vi "Lognormal Moments.vi"(9 "c":dbl=0.6, 10 "b":dbl=1.0) -> (0 "error":i32, 2 "variance":dbl=0.6211037960835473, 3 "mean":dbl=1.1972173631218102)   [LabVIEW 2017, in "NI_Gmath.lvlib"]
doc: "Returns the expected mean and variance of the random variate X, where X describes the selected distribution type. You must manually select the polymorphic instance to use."
uses:
  NI_Gmath.lvlib
  st_error_code.ctl
panel:
  # "Lognormal Moments"
  # "median (scale)"
  # "standard dev (shape)"
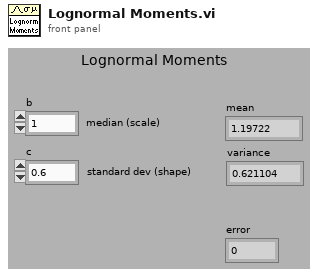
[diagram p1: front panel]
types:
  T1 = typedef "NI_Gmath.lvlib/st_error_code.ctl" = i32
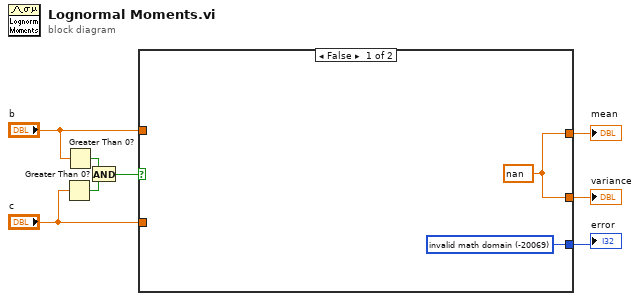
[diagram p0: block diagram]
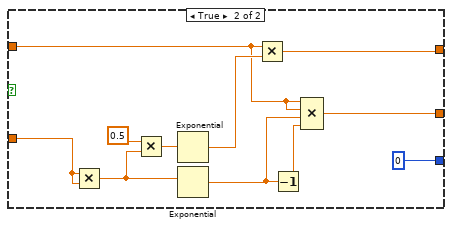
[diagram p2: hidden frame]
diagram:
  n1 = Greater Than 0?(x="c") -> (x > 0?=w7:bool)
  n2 = Greater Than 0?(x="b") -> (x > 0?=w8:bool)
  n3 = And(x=w8, y=w7) -> (x .and. y?=w6:bool)
  n4 = case shown="False" w6 {
    tunnel: [w10 0 ("invalid math domain")] -> w1
    tunnel: [w9 w20] -> w3
    tunnel: [w9 w14] -> w2
    tunnel: "b" -> [_ w17]
    tunnel: "c" -> [_ w18]
    frame False {
      w10 = T1 -20069 items=["invalid math domain"=-20069, "Fourier interpolation size m >= n"=-20070, "empty array"=-20003] ("stat interp error code")
      w9 = nan
    }
    frame True {
      n5 = Multiply(x=w18, y=w18) -> (x*y=w12:dbl)
      n6 = Multiply(x=0.5 ("value"), y=w12) -> (x*y=w11:dbl)
      n7 = Exponential(1:w11) -> (0:w19:dbl)
      n8 = Exponential(1:w12) -> (0:w16:dbl)
      n9 = Multiply(x=w17, y=w19) -> (x*y=w20:dbl)
      n10 = Decrement(x=w16) -> (x-1=w15:dbl)
      n11 = Compound Arithmetic op=MULTIPLY(w17, w17, w16, w15) -> (w14:dbl)
    }
  }
  "mean" <- w3
  "error" <- w1
  "variance" <- w2
